vi "Accelerometer Calibrate.vi"(2 "filter coefficient":dbl=0.02, 3 "sensitivity (raw)":dbl=287.0, 4 "bias (raw)":dbl=1372.0, 5 "raw acceleration":i32[](array[numeric])=[0, 0, 0]) -> (1 "calibrated accelerometer":T1 {"z axis (g)" format="%.3f"; "y axis (g)" format="%.3f"; "x axis (g)" format="%.3f"})   [LabVIEW 2013]
doc: "Calibrate an accelerometer according to a linear model (bias and sensitivity), orientation correction, and lowpass filtering."
uses:
  Accelerometer.ctl
  <vilib>/imath/engines/lvmath2/RunTimeEngine/ErrorHandling/NIMS_Finalize Error.vi
  <vilib>/imath/engines/lvmath2/RunTimeEngine/ArithmeticOperatorToken/NIMS_ArithmeticOperator_plus.vi
  <instcachedir>/0/NIMS_ArithmeticOperator_plus_BB26BEB6C94D4F9C98ECAA4B91B56DD6.lvgen/NIMS_ArithmeticOperator_plus_BB26BEB6C94D4F9C98ECAA4B91B56DD6_004.vi
  <vilib>/imathl/engines/lvmath/Functions/Error Handling/Create Error.vi
  <vilib>/imath/engines/lvmath2/RunTimeEngine/NodeEndStatement/NIMS_NodeEndStatement_Output.vi
  <instcachedir>/0/NIMS_NodeEndStatement_Output_53EC0D466D134D7ABD903AC30B43404B.lvgen/NIMS_NodeEndStatement_Output_53EC0D466D134D7ABD903AC30B43404B_005.vi
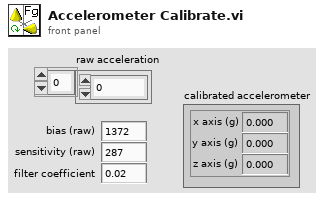
[diagram p1: front panel]
types:
  T1 = typedef "Accelerometer.ctl" = cluster{"x axis (g)":dbl, "y axis (g)":dbl, "z axis (g)":dbl}
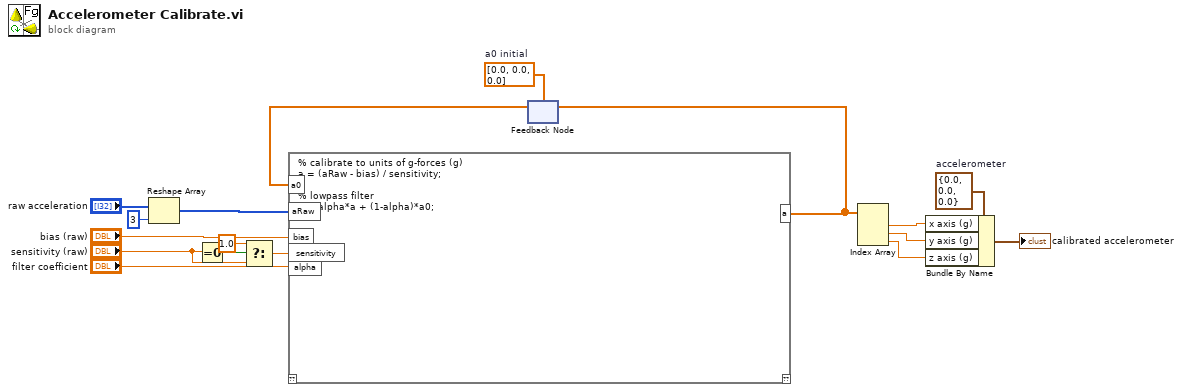
[diagram p0: block diagram]
diagram:
  w7 = dbl[] [0.0, 0.0, 0.0]  # a0 initial
  w16 = T1 {"x axis (g)"=0.0, "y axis (g)"=0.0, "z axis (g)"=0.0}  # accelerometer
  n1 = Reshape Array("raw acceleration", 3 ("dimension size")) -> (w13:i32[])
  n2 = Equal To 0?(x="sensitivity (raw)") -> (x = 0?=w6:bool)
  n3 = Select(t=1.0, s=w6, f="sensitivity (raw)") -> (s? t:f=w4:dbl)
  n4 = feedback #1(w7) -> (w9:dbl[])
  n5 = mathscript code="% calibrate to units of g-forces (g)\na = (aRaw - bias) / sensitivity;\n\n% lowpass filter\na = alpha*a + (1-alpha)*a0;"("aRaw"=w13, "alpha"="filter coefficient", "bias"="bias (raw)", "sensitivity"=w4, "a0"=w9) -> ("a"=w8:dbl[])  [unwired: 1 in, 1 out]
  n6 = feedback-in #1(w8) -> ()
  n7 = Index Array(array=w8) -> (element #1=w12:dbl, element #2=w11:dbl, element #3=w10:dbl)  [unwired: 3 in]
  n8 = Bundle By Name(cluster=w16, "x axis (g)"=w12, "y axis (g)"=w11, "z axis (g)"=w10) -> (→"calibrated accelerometer":T1)
